vi "Open.vi"(8 "error in (no error)":errorcluster, 11 "MelsecTCP in":refnum<class "InovanceTCP.lvclass">) -> (0 "error out":errorcluster, 3 "MelsecTCP out":refnum<class "InovanceTCP.lvclass">)   [LabVIEW 2020, in "HslCommunication.lvlib" / "InovanceTCP.lvclass"]
uses:
  InovanceTCP.lvclass
  D:/Git/Labview-Libraries/Libraries/HslCommunication/Abstract PLC Controler/Abstract PLC Controler.lvclass
  EventLogger.lvlibp/1abvi3w/vi.lib/gpm_packages/@cs/event-logger/Source/Composed Log/Types/Log Level.ctl
  Abstract PLC Controler/Abstract PLC Controler.lvclass/Abstract PLC Controler.ctl
  D:/Git/Labview-Libraries/Libraries/HslCommunication/_Dependenciecs/HslCommunication.dll
  _Dependenciecs/HslCommunication.dll
  InovanceTCP.lvclass/InovanceTCP.ctl
  Read ipAddress.vi
  Read port.vi
  Abstract PLC Controler/Abstract PLC Controler.lvclass
  EventLogger.lvlibp/Logger.lvclass
  EventLogger.lvlibp/1abvi3w/vi.lib/gpm_packages/@cs/event-logger/Source/Composed Log/Composed Log.lvlib
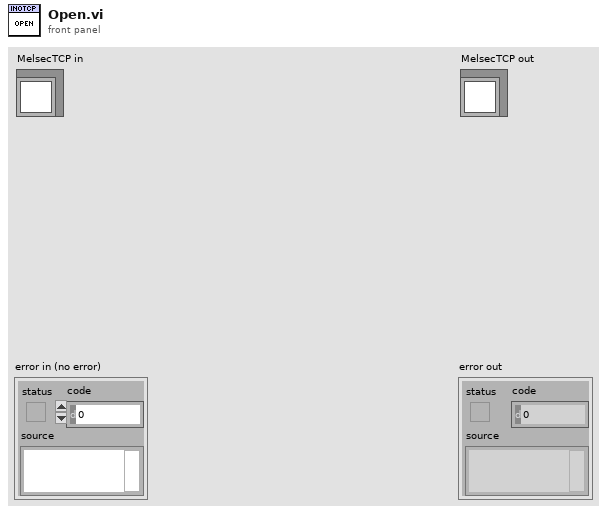
[diagram p1: front panel]
types:
  T1 = typedef "EventLogger.lvlibp/Composed Log.lvlib/Log Level.ctl" = enum16{"Debug", "Info", "Warning", "Error", "Critical"}
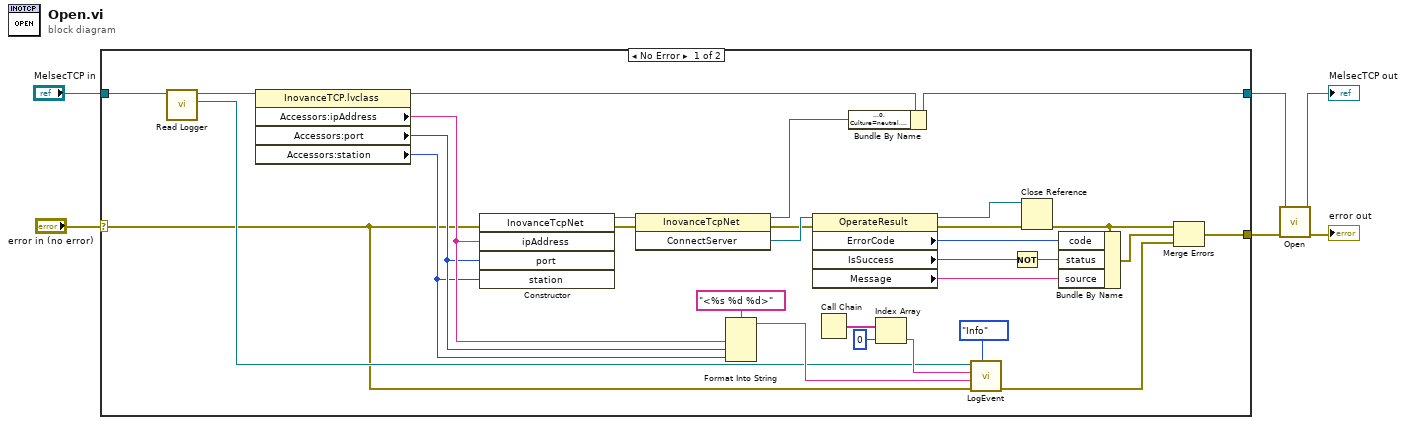
[diagram p0: block diagram]
diagram:
  n1 = case shown="No Error" "error in (no error)" {
    selector: "error in (no error)" -> [w9 w38]
    tunnel: "MelsecTCP in" -> [w36 w37]
    tunnel: [w35 w37] -> w2
    tunnel: [w29 w38] -> w4
    frame No Error {
      n2 = call "Read Logger.vi"("Abstract PLC Controler in"=w36) -> ("EventLogger.lvlibp:Logger.lvclass"=w10:refnum<class "Logger.lvclass">, "Abstract PLC Controler out"=w19:refnum<class "InovanceTCP.lvclass">)  [unwired: 9 in]
      n3 = property class="InovanceTCP.lvclass"(reference=w19) -> (reference out=w20:refnum<class "InovanceTCP.lvclass">, "Accessors:ipAddress"=w16:string, "Accessors:port"=w15:i32, "Accessors:station"=w14:u8)  [unwired: 1 in, 1 out]
      n4 = constructor class="InovanceTcpNet"(error in=w9, "ipAddress"=w16, "port"=w15, "station"=w14) -> (reference out=w24:refnum<k24>, error out=w23:errorcluster)  [unwired: 2 in, 4 out]
      n5 = invoke class="InovanceTcpNet" method="ConnectServer"(reference=w24, error in=w23) -> (reference out=w21:refnum<k24>, error out=w26:errorcluster, "ConnectServer"=w28:refnum<k24>)  [unwired: 1 in]
      n6 = Format Into String(format string="<%s %d %d>", w16, w15, w14) -> (resulting string=w12:string)  [unwired: 2 in, 1 out]
      n7 = property class="OperateResult"(reference=w28, error in=w26) -> (reference out=w27:refnum<k24>, error out=w25:errorcluster, "ErrorCode"=w32:i32, "IsSuccess"=w22:bool, "Message"=w30:string)
      n8 = Call Chain() -> (call chain=w18:string[])
      n9 = Bundle By Name(cluster=w20, "reference"=w21) -> (w35:refnum<class "InovanceTCP.lvclass">)
      n10 = Index Array(array=w18, index=0) -> (element=w11:string)
      n11 = call "LogEvent.vi"("Event Level"=Log_Level."Info", "error in (no error)"=w9, "Data To Log"=w12, "SourceID"=w11, "Logger in"=w10) -> ("error out"=w8:errorcluster)  [unwired: 5 in, 1 out]
      n12 = Not(x=w22) -> (.not. x?=w31:bool)
      n13 = Close Reference(reference=w27, error in (no error)=w25) -> (error out=w33:errorcluster)
      n14 = Bundle By Name(cluster=w33, "code"=w32, "status"=w31, "source"=w30) -> (w34:errorcluster)
      n15 = Merge Errors(w33, w34, w8) -> (w29:errorcluster)
    }
    frame Error {
    }
  }
  n16 = call-parent "Open.vi"("error in (no error)"=w4, "MelsecTCP in"=w2) -> ("error out"=→"error out":errorcluster, "MelsecTCP out"=→"MelsecTCP out":refnum<class "InovanceTCP.lvclass">)  [unwired: 8 in]
